vi "CAN_Command Motor.vi"(0 "Write":refnum<k21>, 1 "Read":refnum<k21>, 4 "ID Request":string="18DA55F2", 5 "Numeric Request":u32 format="%x", 6 "ID Response":string="18DAF255", 16 "CAN Command":string) -> (2 "Data String 10":string, 3 "Data String 5":string, 7 "Data String 2":string, 8 "Data String 9":string, 9 "Data String 7":string, 10 "Data String 4":string, 11 "Data String 3":string, 12 "Data String 8":string, 13 "Timestamp":timestamp, 14 "Read out":refnum<k21>, 15 "Write out":refnum<k21>, 17 "Data String 6":string, 18 "ID String":string, 19 "Data String":string)   [LabVIEW 2023]
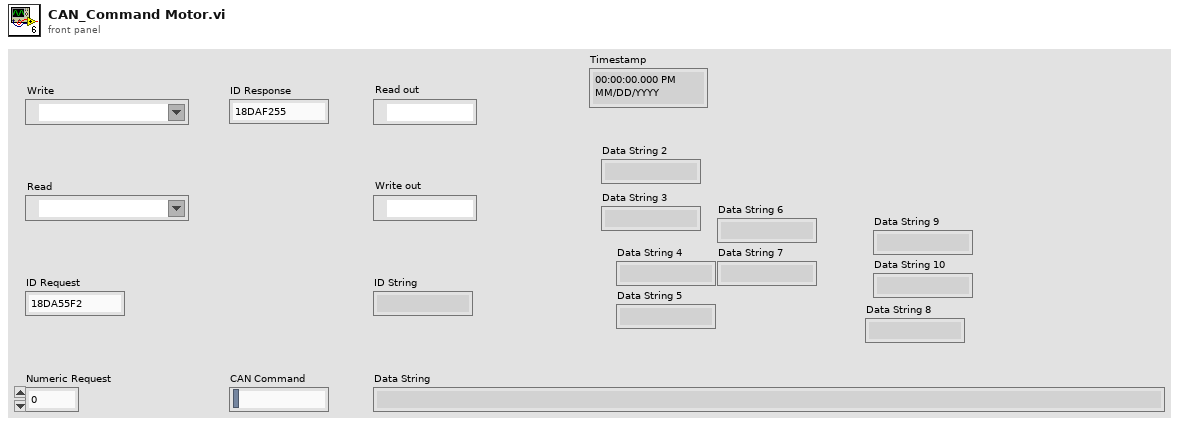
[diagram p1: front panel]
types:
  T1 = typedef "XNET Frame CAN.ctl" = cluster{"timestamp":timestamp, "payload":u8[], "identifier":u32, "type":T2, "extended?":bool, "echo?":bool}
  T2 = typedef "XNET Frame Type CAN.ctl" = u8
  T3 = cluster{"data[0]":T1, "data[1]":T1, "data[2]":T1, "data[3]":T1, "data[4]":T1, "data[5]":T1, "data[6]":T1, "data[7]":T1, "data[8]":T1}
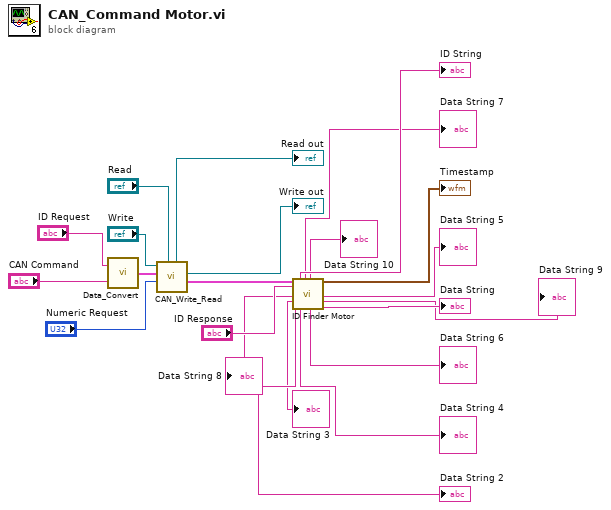
[diagram p0: block diagram]
diagram:
  n1 = call "Data_Convert.vi"("string"="CAN Command", "ID"="ID Request") -> ("CAN frame"=w19:T1)
  n2 = call "CAN_Write_Read.vi"("Read In"="Read", "Numeric Request"="Numeric Request", "CAN frame"=w19, "Write In"="Write") -> ("cluster"=w20:T3, "Write Out"=→"Write out":refnum<k21>, "Read Out"=→"Read out":refnum<k21>)  [unwired: 1 in, 2 out]
  n3 = call "ID Finder Motor.vi"("cluster"=w20, "ID ESPERADO STRING"="ID Response") -> ("Data String 8"=→"Data String 8":string, "Data String 3"=→"Data String 3":string, "Data String 2"=→"Data String 2":string, "ID String"=→"ID String":string, "Data String 4"=→"Data String 4":string, "Data String 7"=→"Data String 7":string, "Data String 10"=→"Data String 10":string, "Data String 6"=→"Data String 6":string, "Timestamp"=→"Timestamp":timestamp, "Data String 5"=→"Data String 5":string, "Data String 9"=→"Data String 9":string, "Data String"=→"Data String":string)  [unwired: 3 in, 3 out]
